vi "SeparaMemoriaSetDadosInversor.vi"(8 "error in":errorcluster) -> (0 "error out":errorcluster, 3 "Memorias":T1(array[cluster]))   [LabVIEW 2019]
uses:
  TelaConfig/Configuracao.Variaveis.vi
  TelaParametrosTeste/VariaveisParametros.vi
  VariaveisMedicao.vi
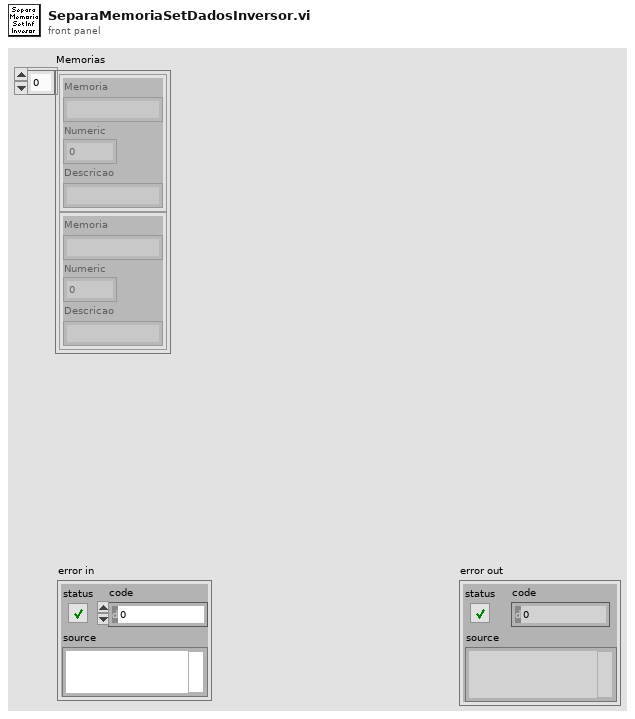
[diagram p1: front panel]
types:
  T1 = cluster{"Memoria":string, "Numeric":dbl, "Descricao":string}[]
  T2 = enum16{"None", "Continua", "Senoidal", "Quadrada"}
  T3 = cluster{"Memoria":string, "Numeric":dbl, "Descricao":string}
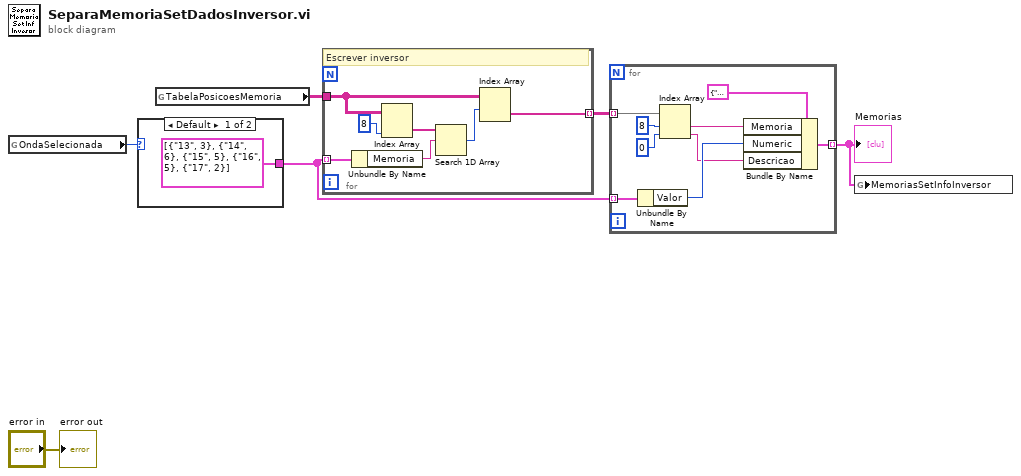
[diagram p0: block diagram]
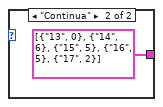
[diagram p2: hidden frame]
diagram:
  n1 = global read "VariaveisParametros.vi" "OndaSelecionada"() -> (w3:T2)
  n2 = case shown="Default" w3 {
    tunnel: [cluster{"Memoria":string, "Valor":i32}[] [{"Memoria"="13", "Valor"=3}, {"Memoria"="14", "Valor"=6}, {"Memoria"="15", "Valor"=5}, {"Memoria"="16", "Valor"=5}, {"Memoria"="17", "Valor"=2}] ("Array") cluster{"Memoria":string, "Valor":i32}[] [{"Memoria"="13", "Valor"=0}, {"Memoria"="14", "Valor"=6}, {"Memoria"="15", "Valor"=5}, {"Memoria"="16", "Valor"=5}, {"Memoria"="17", "Valor"=2}] ("Array")] -> w2
    frame Default {
    }
    frame "Continua" {
    }
  }
  n3 = global read "Configuracao.Variaveis.vi" "TabelaPosicoesMemoria"() -> (w5:string[][])
  n4 = for {
    tunnel: w5 -> [w12]
    tunnel: [w11] -> w6 mode=indexing
    tunnel: w2 -> [w10] mode=indexing
    # "Escrever inversor"
    n5 = Unbundle By Name(w10) -> ("Memoria"=w9:string)
    n6 = Index Array(array=w12, index (col)=8 ("disabled index (col)")) -> (element=w13:string[])  [unwired: 1 in]
    n7 = Search 1D Array(1D array=w13, element=w9) -> (index of element=w15:i32)  [unwired: 1 in]
    n8 = Index Array(array=w12, index (row)=w15) -> (element=w11:string[])  [unwired: 1 in]
  }
  n9 = for {
    tunnel: w6 -> [w23] mode=indexing
    tunnel: w2 -> [w22] mode=indexing
    tunnel: [w16] -> w1 mode=indexing
    n10 = Unbundle By Name(w22) -> ("Valor"=w19:i32)
    n11 = Index Array(array=w23, index #1=8 ("index"), index #2=0 ("index")) -> (element #1=w20:string, element #2=w17:string)
    n12 = Bundle By Name(cluster=T3 {"Memoria"="", "Numeric"=0.0, "Descricao"=""} ("Cluster"), "Memoria"=w20, "Numeric"=w19, "Descricao"=w17) -> (w16:T3)
  }
  "Memorias" <- w1
  n13 = global write "VariaveisMedicao.vi" "MemoriasSetInfoInversor"(w1) -> ()
  "error out" <- "error in"
